vi "Resideo Gas Valve - Get Data.vi"(8 "error in (no error)":errorcluster, 11 "VISA resource name":refnum<visa-resource-name>) -> (0 "error out":errorcluster, 2 "Vesta Data Output":T1, 3 "Vesta Data":string[][](array[string]))   [LabVIEW 2020]
uses:
  Type Definitions/Vesta Info.ctl
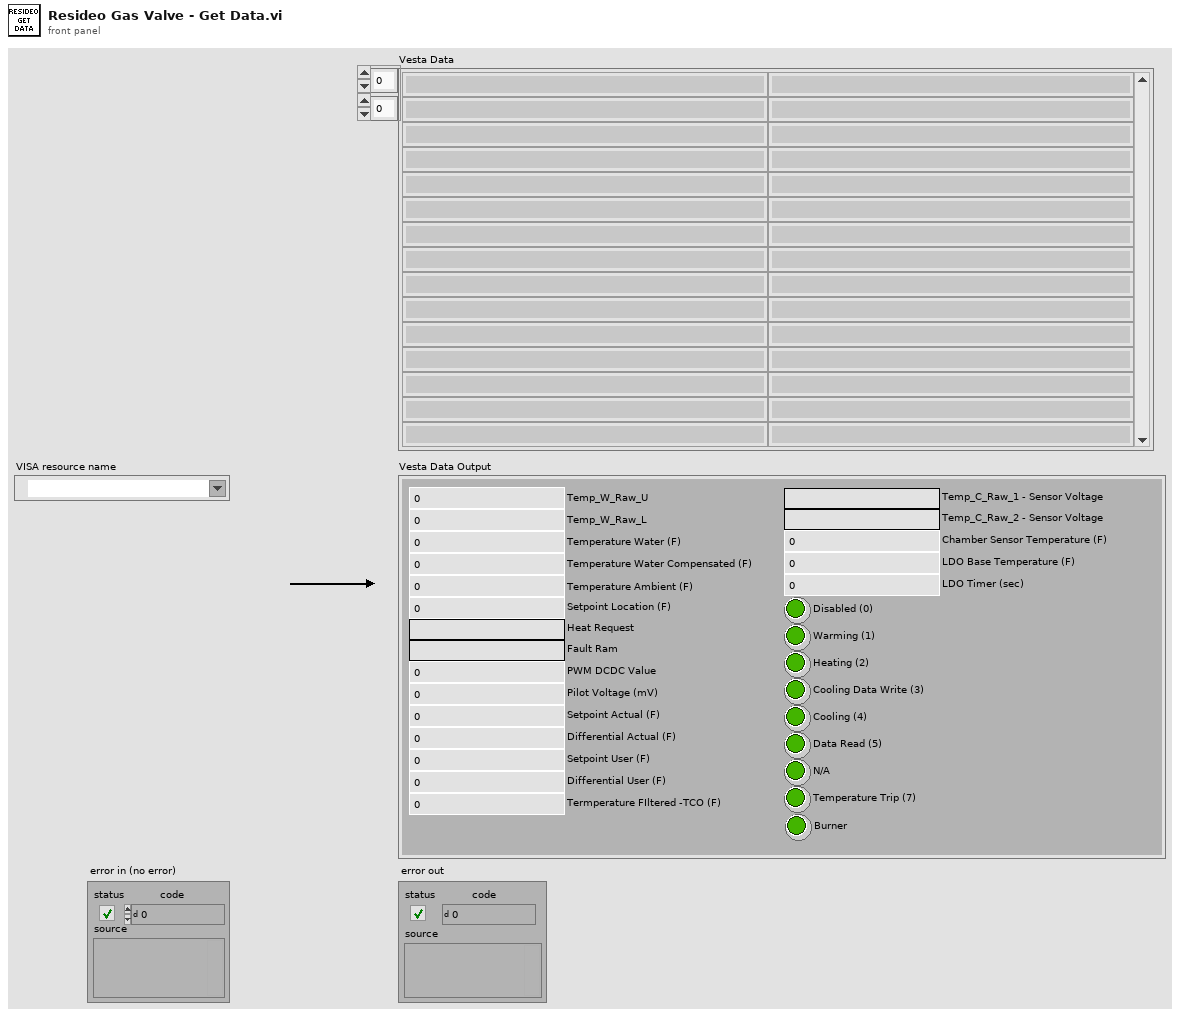
[diagram p1: front panel]
types:
  T1 = typedef "Vesta Info.ctl" = cluster{"Temp_W_Raw_U":u16, "Temp_W_Raw_L":u16, "Temperature Water (F)":dbl, "Temperature Water Compensated (F)":dbl, "Temperature Ambient (F)":dbl, "Setpoint Location (F)":dbl, "Heat Request":string, "Fault Ram":string, "PWM DCDC Value":u16, "Pilot Voltage (mV)":dbl, "Setpoint Actual (F)":dbl, "Differential Actual (F)":dbl, "Setpoint User (F)":dbl, "Differential User (F)":dbl, "Termperature FIltered -TCO (F)":dbl, "Temp_C_Raw_1 - Sensor Voltage":string, "Temp_C_Raw_2 - Sensor Voltage":string, "Chamber Sensor Temperature (F)":dbl, "LDO Base Temperature (F)":dbl, "LDO Timer (sec)":i16, "Disabled (0)":bool, "Warming (1)":bool, "Heating (2)":bool, "Cooling Data Write (3)":bool, "Cooling (4)":bool, "Data Read (5)":bool, "N/A":bool, "Temperature Trip (7)":bool, "Burner":bool}
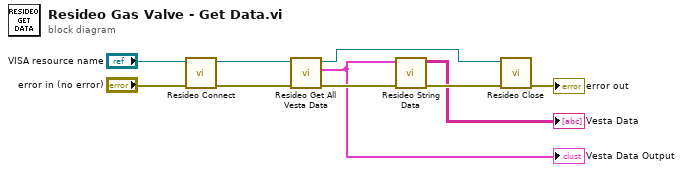
[diagram p0: block diagram]
diagram:
  n1 = call "Resideo Connect.vi"("error in (no error)"="error in (no error)", "VISA Refnum in"="VISA resource name") -> ("error out"=w9:errorcluster, "Modbus Master out"=w7:refnum<class "Modbus Master.lvclass">)  [unwired: 8 in]
  n2 = call "Resideo Get All Vesta Data.vi"("error in (no error)"=w9, "Modbus Master in"=w7) -> ("error out"=w3:errorcluster, "Vesta Data Output"=w1:T1, "Modbus Master out"=w6:refnum<class "Modbus Master.lvclass">)  [unwired: 7 in]
  "Vesta Data Output" <- w1
  n3 = call "Resideo String Data.vi"("error in (no error)"=w3, "Vesta LDO"=w1) -> ("error out"=w4:errorcluster, "Vesta Data"=→"Vesta Data":string[][])  [unwired: 7 in, 1 out]
  n4 = call "Resideo Close.vi"("error in (no error)"=w4, "Modbus Master in"=w6) -> ("error out"=→"error out":errorcluster)  [unwired: 9 in]
